vi "ParseBusMonitorTxtLog.vi"(8 "error in (no error)":errorcluster, 10 "Path":path=path "C:/LVLibrary/XNET/XCP_DaqDtoID/XCP_DaqDtoId/ECUMCLog/BusMonitorLog.txt", 11 "DAQList in":refnum<class "DAQList.lvclass">) -> (0 "error out":errorcluster, 2 "CAN Frames":T1[](array[typedef]) {"payload" format="%x"; "timestamp" format="%<%.7X\n%x>T"; "type" items=["CAN Data"=0, "CAN Remote"=1, "CAN Bus Error"=2, "CAN 2.0 Data"=8, "CAN FD Data"=16, "CAN FD+BRS Data"=24, "J1939 Data"=192, "Delay"=224, "Log Trigger"=225, "Start Trigger"=226]; "identifier" format="%x"}, 3 "DAQList out":refnum<class "DAQList.lvclass">)   [LabVIEW 2019]
uses:
  DAQList.lvclass
  <vilib>/xnet/xnet.llb/XNET Frame CAN.ctl
  <vilib>/xnet/xnet.llb/XNET Frame Type CAN.ctl
  <vilib>/Utility/file.llb/Read Delimited Spreadsheet (string).vi
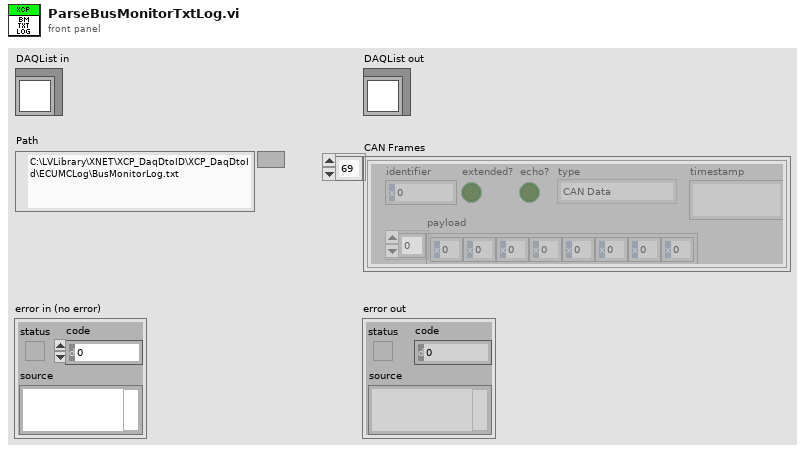
[diagram p1: front panel]
types:
  T1 = typedef "XNET Frame CAN.ctl" = cluster{"timestamp":timestamp, "payload":u8[], "identifier":u32, "type":T2, "extended?":bool, "echo?":bool}
  T2 = typedef "XNET Frame Type CAN.ctl" = u8
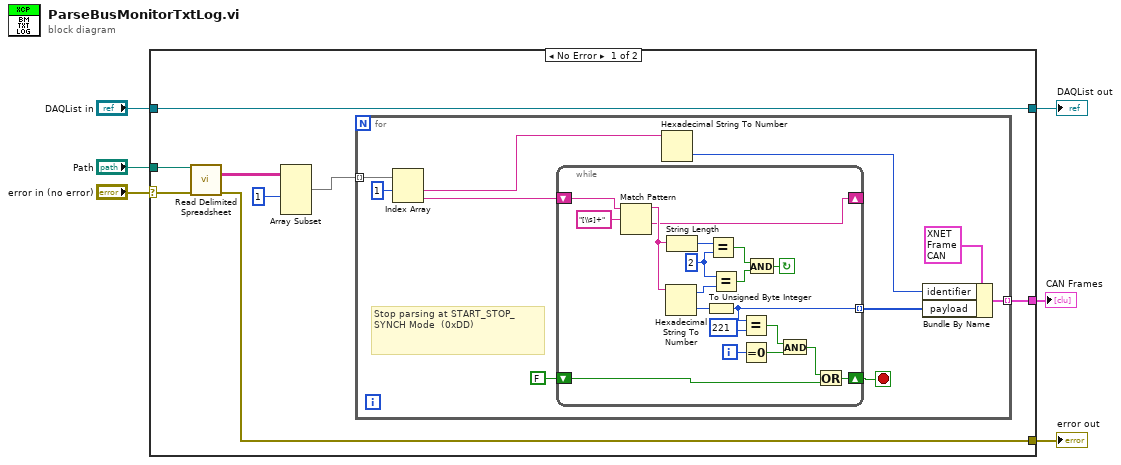
[diagram p0: block diagram]
diagram:
  n1 = case shown="No Error" "error in (no error)" {
    selector: "error in (no error)" -> [w12 w45]
    tunnel: [w11 w45] -> w5
    tunnel: [w14 w44] -> w3
    tunnel: "DAQList in" -> [w14 w44]
    tunnel: "Path" -> [w13 _]
    tunnel: [w7 _] -> w1
    frame No Error {
      n2 = call-poly <vilib>:"Read Delimited Spreadsheet.vi"("file path (dialog if empty)"=w13, "error in (no error)"=w12) -> ("all rows"=w9:string[][], "error out"=w11:errorcluster)  [unwired: 8 in, 4 out]
      n3 = Array Subset(array=w9, index (row)=1 ("index")) -> (w8:string[][])  [unwired: 3 in]
      n4 = for {
        tunnel: w8 -> [w16] mode=indexing
        tunnel: [w22] -> w7 mode=indexing
        stop <- w17 stop-if-true
        # "Stop parsing at START_STOP_SYNCH Mode  (0xDD)"
        n5 = Index Array(array=w16, index #1=1 ("index")) -> (element #1=w20:string, element #2=w15:string)  [unwired: 1 in]
        n6 = while {
          shift-right: [w34] -> _
          shift-left: w15 -> [w43]
          tunnel: [w31] -> w23 mode=indexing
          shift-right: [w26] -> w17
          shift-left: FALSE -> [w25]
          i -> [w32]
          stop <- w35 continue-if-true
          w39 = 2 ("y")
          n7 = Match Pattern(string=w43, regular expression="[\\s]+") -> (before substring=w40:string, after substring=w34:string)  [unwired: 1 in, 2 out]
          n8 = Hexadecimal String To Number(string=w40) -> (offset past number=w38:i32, number=w33:u32)  [unwired: 2 in]
          n9 = String Length(string=w40) -> (length=w41:i32)
          n10 = To Unsigned Byte Integer(number=w33) -> (unsigned 8bit integer=w31:u8)
          n11 = Equal?(x=w41, y=w39) -> (x = y?=w37:bool)
          n12 = Equal?(x=w39, y=w38) -> (x = y?=w36:bool)
          n13 = Equal?(x=w31, y=u8 221 ("unsigned 8bit integer")) -> (x = y?=w29:bool)
          n14 = Equal To 0?(x=w32) -> (x = 0?=w28:bool)
          n15 = And(x=w37, y=w36) -> (x .and. y?=w35:bool)
          n16 = And(x=w29, y=w28) -> (x .and. y?=w27:bool)
          n17 = Or(x=w27, y=w25) -> (x .or. y?=w26:bool)
        }
        n18 = Hexadecimal String To Number(string=w20) -> (number=w19:u32)  [unwired: 2 in, 1 out]
        n19 = Bundle By Name(cluster=T1 {"timestamp"=timestamp(0 s since 1904-01-01), "payload"=[], "identifier"=0, "type"=0, "extended?"=FALSE, "echo?"=FALSE} ("CAN frame"), "identifier"=w19, "payload"=w23) -> (w22:T1)
      }
    }
    frame Error {
    }
  }
  "error out" <- w5
  "DAQList out" <- w3
  "CAN Frames" <- w1
